vi "CRC.vi"(1 "Data":u8[](array[numeric])) -> (0 "Data + CRC":u8[](array[numeric]))   [LabVIEW 2022 SP3]
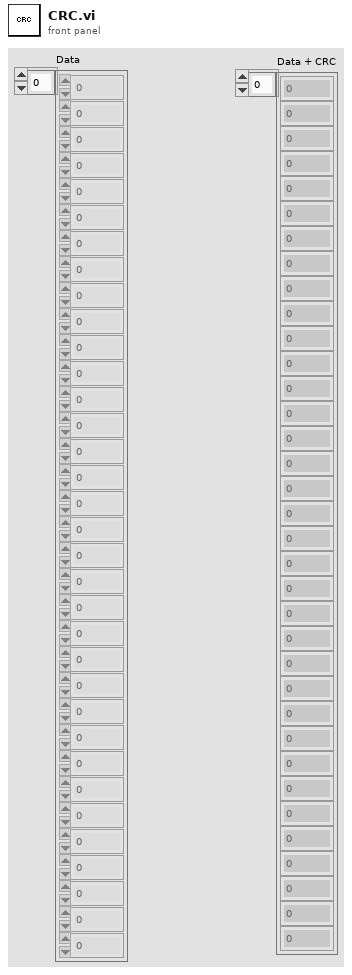
[diagram p1: front panel]
types:
  T1 = cluster{" Polynomial * 2[0]":u8, " Polynomial * 2[1]":u8, " Polynomial * 2[2]":u8}
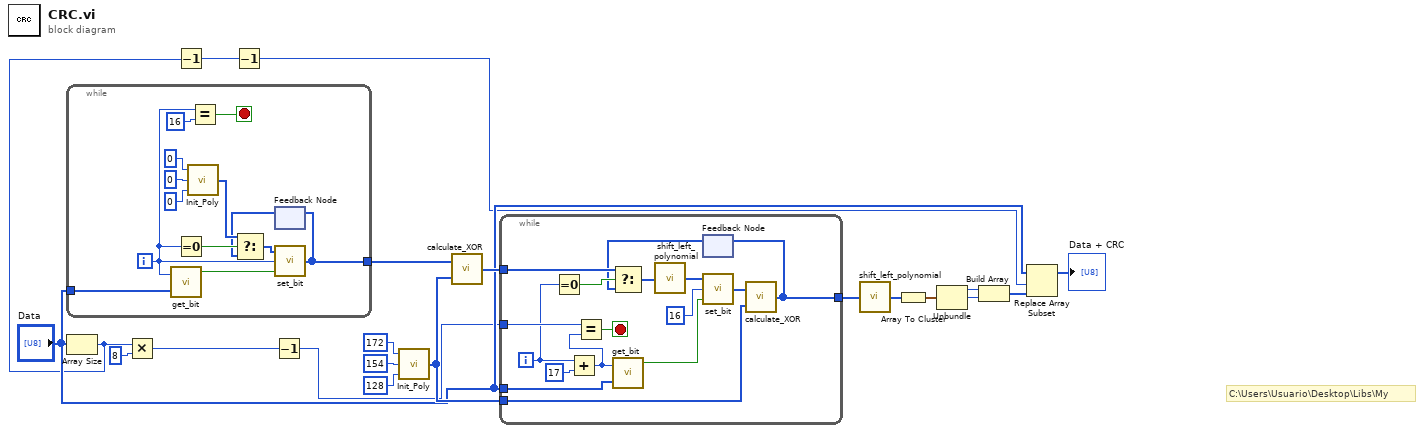
[diagram p0: block diagram]
diagram:
  # "C:\\Users\\Usuario\\Desktop\\Libs\\My"
  n1 = while {
    tunnel: [w22] -> w20
    tunnel: "Data" -> [w21]
    i -> [w24]
    stop <- w32 stop-if-true
    n2 = call "get_bit.vi"("Position"=w24, "INFO"=w21) -> ("Bit_Value"=w31:bool)  [unwired: 2 out]
    n3 = Equal To 0?(x=w24) -> (x = 0?=w27:bool)
    n4 = call "Init_Poly.vi"("2"=u8 0, "1"=u8 0, "0"=u8 0) -> ("POLY"=w26:u8[])
    n5 = Equal?(x=w24, y=u16 16) -> (x = y?=w32:bool)
    n6 = feedback #1() -> (w25:u8[])  [unwired: 1 in]
    n7 = Select(t=w26, s=w27, f=w25) -> (s? t:f=w23:u8[])
    n8 = call "set_bit.vi"("State"=w31, "Position"=w24, "Array"=w23) -> ("Array 2"=w22:u8[])
    n9 = feedback-in #1(w22) -> ()
  }
  n10 = Array Size(array="Data") -> (size(s)=w2:i32)
  n11 = Multiply(x=w2, y=8) -> (x*y=w15:i32)
  n12 = Decrement(x=w2) -> (x-1=w3:i32)
  n13 = Decrement(x=w3) -> (x-1=w1:i32)
  n14 = Decrement(x=w15) -> (x-1=w10:i32)
  n15 = call "Init_Poly.vi"("2"=u8 128, "1"=u8 154, "0"=u8 172) -> ("POLY"=w13:u8[])
  n16 = call "calculate_XOR.vi"("Divisor"=w13, "Initial Poly"=w20) -> ("Array"=w14:u8[])
  n17 = while {
    tunnel: w10 -> [w48]
    tunnel: w14 -> [w46]
    tunnel: "Data" -> [w42]
    tunnel: w13 -> [w38]
    tunnel: [w35] -> w12
    i -> [w44]
    stop <- w49 stop-if-true
    n18 = Equal To 0?(x=w44) -> (x = 0?=w47:bool)
    n19 = Add(x=w44, y=17) -> (x+y=w34:i32)
    n20 = Equal?(x=w48, y=w34) -> (x = y?=w49:bool)
    n21 = call "get_bit.vi"("Position"=w34, "INFO"=w42) -> ("Bit_Value"=w40:bool)  [unwired: 2 out]
    n22 = feedback #2() -> (w36:u8[])  [unwired: 1 in]
    n23 = Select(t=w46, s=w47, f=w36) -> (s? t:f=w45:u8[])
    n24 = call "shift_left_polynomial.vi"("Polynomial"=w45) -> ("Polynomial * 2"=w41:u8[])
    n25 = call "set_bit.vi"("State"=w40, "Position"=u16 16, "Array"=w41) -> ("Array 2"=w37:u8[])
    n26 = call "calculate_XOR.vi"("Divisor"=w38, "Initial Poly"=w37) -> ("Array"=w35:u8[])
    n27 = feedback-in #2(w35) -> ()
  }
  n28 = call "shift_left_polynomial.vi"("Polynomial"=w12) -> ("Polynomial * 2"=w9:u8[])
  n29 = Array To Cluster(array=w9) -> (cluster=w8:T1)
  n30 = Unbundle(w8) -> ("Polynomial * 2[0]"=w7:u8, "Polynomial * 2[1]"=w6:u8)  [unwired: 1 out]
  n31 = Build Array(w7, w6) -> (w5:u8[])
  n32 = Replace Array Subset(array="Data", new element=w5, index=w1) -> (→"Data + CRC":u8[])
